vi "timing_data_to_boolean_array.vi"(2 "end time [s]":dbl=1.0, 3 "start time [s]":dbl, 4 "overall length [s]":dbl=1000.0) -> (0 "boolean timing array":bool[](array[boolean]))   [LabVIEW 2011]
doc: "Creates a boolean array based on the timing info send in. Used to display a digital waveform graph to visualize the timing info recieved and send to the Standford Research Systems DG645 Delay Generator. \nWorks only in combination with values in seconds. Can be used for any timing value in combination with the standardize array vi."
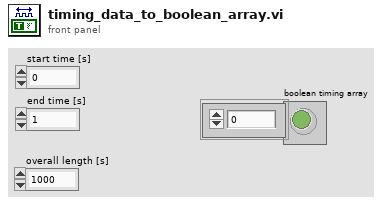
[diagram p1: front panel]
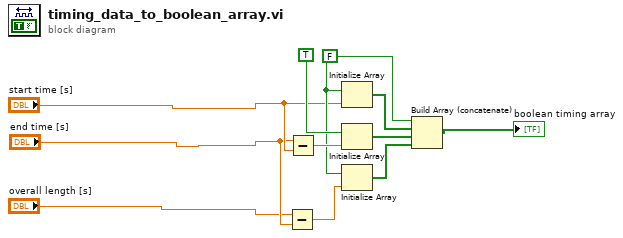
[diagram p0: block diagram]
diagram:
  w5 = FALSE
  n1 = Subtract(x="overall length [s]", y="end time [s]") -> (x-y=w10:dbl)
  n2 = Subtract(x="end time [s]", y="start time [s]") -> (x-y=w6:dbl)
  n3 = Initialize Array(w5, "start time [s]") -> (w11:bool[])
  n4 = Initialize Array(TRUE, w6) -> (w7:bool[])
  n5 = Initialize Array(w5, w10) -> (w9:bool[])
  n6 = Build Array (concatenate)(w5, w11, w7, w9) -> (→"boolean timing array":bool[])
